vi "single shot DC V read.vi"(6 "error in":errorcluster, 8 "Clear":bool=TRUE, 9 "DAQmx Physical Channel":tag="Dev1/ai0") -> (0 "error out":errorcluster, 3 "data":dbl format="%0.2f")   [LabVIEW 2013]
doc: "This one shot vi measures a single shot voltage on a defined analog channel\n\nMatt Strader\nPaul K Dixon\nPhysics 350\nCSUSB Physics"
uses:
  <vilib>/DAQmx/read.llb/DAQmx Read (Analog DBL 1Chan 1Samp).vi
  <vilib>/DAQmx/create/channels.llb/DAQmx Create Channel (AI-Voltage-Basic).vi
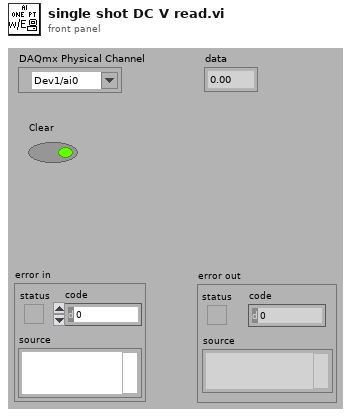
[diagram p1: front panel]
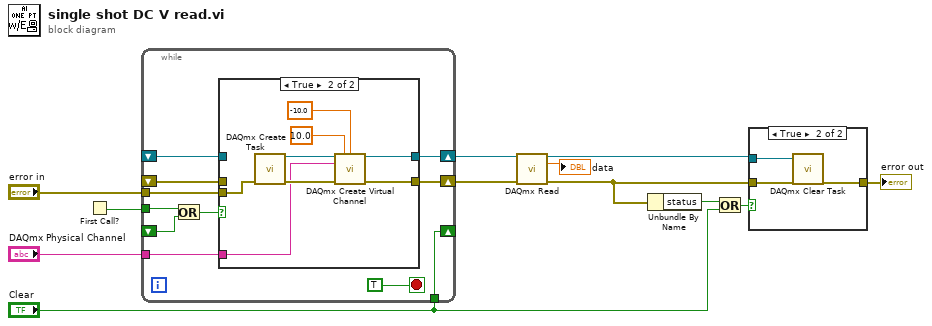
[diagram p0: block diagram]
diagram:
  n1 = First Call?() -> (First Call?: T/F=w8:bool)
  n2 = while "InitWhileLoop" {
    tunnel: "error in" -> [w21]
    shift-right: [w20] -> _
    shift-left: _ -> [w19]
    tunnel: "Clear" -> [w20]
    tunnel: w8 -> [w17]
    shift-right: [w23] -> w5
    shift-left: _ -> [w16]
    shift-right: [w15] -> w6
    shift-left: _ -> [w14]
    tunnel: "DAQmx Physical Channel" -> [w13]
    stop <- TRUE stop-if-true
    n3 = Or(x=w17, y=w19) -> (x .or. y?=w18:bool)
    n4 = case "InitCaseStructure" shown="True" w18 {
      tunnel: [w25 w28] -> w23
      tunnel: w21 -> [_ w31]
      tunnel: w16 -> [w25 _]
      tunnel: [w24 w29] -> w15
      tunnel: w14 -> [w24 _]
      tunnel: w13 -> [_ w30]
      frame False {
      }
      frame True {
        n5 = call <vilib>:"DAQmx Create Task.vi"("error in"=w31) -> ("task out"=w32:refnum<k21>, "error out"=w33:errorcluster)  [unwired: 4 in, 9 out]
        n6 = call-poly <vilib>:"DAQmx Create Virtual Channel.vi"("task in"=w32, "maximum value"=10.0, "minimum value"=-10.0, "physical channels"=w30, "error in"=w33) -> ("task out"=w29:refnum<k21>, "error out"=w28:errorcluster)  [unwired: 4 in, 5 out]
      }
    }
  }
  n7 = call-poly <vilib>:"DAQmx Read.vi"("task/channels in"=w6, "error in"=w5) -> ("task out"=w7:refnum<k21>, "data"=→"data":dbl, "error out"=w4:errorcluster)  [unwired: 1 in, 10 out]
  n8 = Unbundle By Name(w4) -> ("status"=w11:bool)
  n9 = Or(x=w11, y="Clear") -> (x .or. y?=w10:bool)
  n10 = case shown="True" w10 {
    tunnel: [w34 w36] -> w1
    tunnel: w4 -> [w34 w37]
    tunnel: w7 -> [_ w35]
    frame False {
    }
    frame True {
      n11 = call <vilib>:"DAQmx Clear Task.vi"("task in"=w35, "error in"=w37) -> ("error out"=w36:errorcluster)  [unwired: 13 out]
    }
  }
  "error out" <- w1
